vi "Generate Patch Sequence.vi"(8 "Total Number of Frames in a trial":i32, 9 "No of Patches in Cycle":i32, 10 "Current Patch No":i32, 11 "Trial number":i32) -> (0 "sequence for specific trial":i32[](array[numeric]), 2 "Patch Sequence":i32[](array[numeric]))   [LabVIEW 2017]
panel:
  out "size(s)":i32
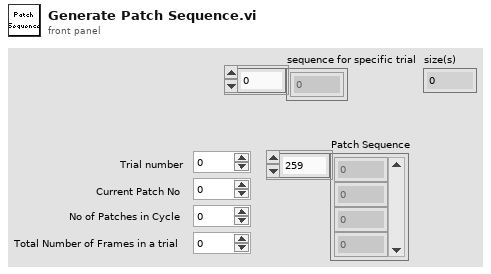
[diagram p1: front panel]
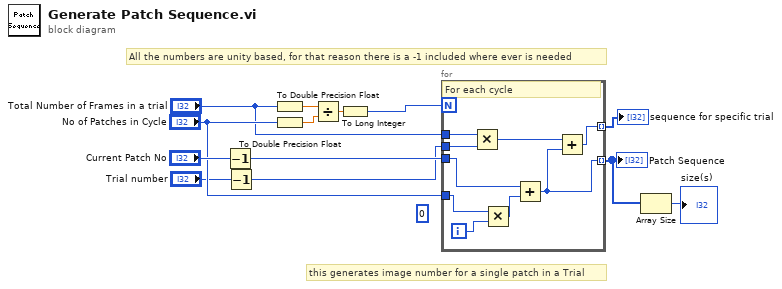
[diagram p0: block diagram]
diagram:
  (unwired) 0 ("No of Patches in Cycle")
  # "this generates image number for a single patch in a Trial"
  # "All the numbers are unity based, for that reason there is a -1 included where ever is needed"
  n1 = Decrement(x="Current Patch No") -> (x-1=w7:i32)
  n2 = Decrement(x="Trial number") -> (x-1=w5:i32)
  n3 = To Double Precision Float(number="Total Number of Frames in a trial") -> (double precision float=w12:dbl)
  n4 = To Double Precision Float(number="No of Patches in Cycle") -> (double precision float=w11:dbl)
  n5 = Divide(x=w12, y=w11) -> (x/y=w13:dbl)
  n6 = To Long Integer(number=w13) -> (32bit integer=w10:i32)
  n7 = for {
    N: w10 -> [_]
    tunnel: w7 -> [w15]
    tunnel: w5 -> [w22]
    tunnel: "No of Patches in Cycle" -> [w17]
    tunnel: [w14] -> w2 mode=indexing
    tunnel: "Total Number of Frames in a trial" -> [w21]
    tunnel: [w19] -> w3 mode=indexing
    i -> [w18]
    # "For each cycle"
    n8 = Multiply(x=w21, y=w22) -> (x*y=w20:i32)
    n9 = Multiply(x=w17, y=w18) -> (x*y=w16:i32)
    n10 = Add(x=w15, y=w16) -> (x+y=w14:i32)
    n11 = Add(x=w20, y=w14) -> (x+y=w19:i32)
  }
  "Patch Sequence" <- w2
  "sequence for specific trial" <- w3
  n12 = Array Size(array=w2) -> (size(s)=→"size(s)":i32)
